vi "Update fgv objectives.vi"(8 "error in (no error)":errorcluster, 11 "Config cluster IN":T1) -> (0 "error out":errorcluster)   [LabVIEW 2017]
uses:
  Typedefs/Calibration config.ctl
  Typedefs/Objective Config.ctl
  Typedefs/Prechirper Cal Config.ctl
  Typedefs/PreChirper constants.ctl
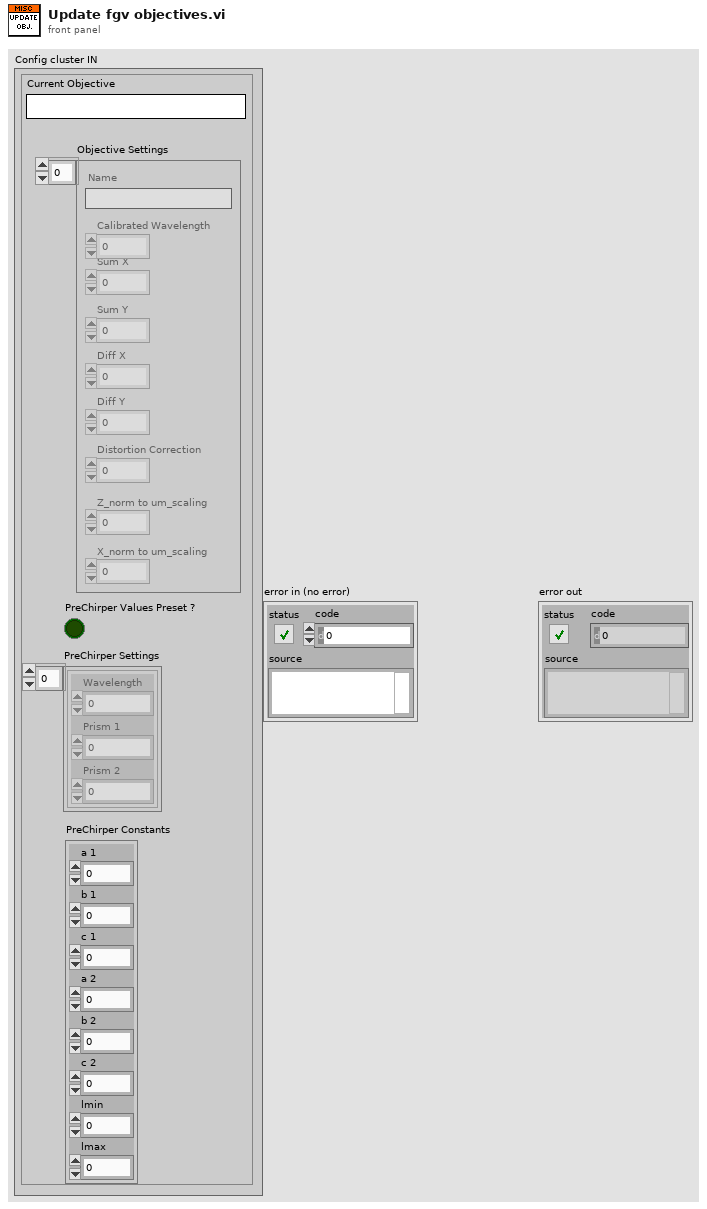
[diagram p1: front panel]
types:
  T1 = typedef "Calibration config.ctl" = cluster{"Current Objective":string, "Objective Settings":T2[], "PreChirper Values Preset ?":bool, "PreChirper Settings":T3[], "PreChirper Constants":T4}
  T2 = typedef "Objective Config.ctl" = cluster{"Name":string, "Sum X":dbl, "Sum Y":dbl, "Diff X":dbl, "Diff Y":dbl, "Distortion Correction":dbl, "Z_norm to um_scaling":dbl, "X_norm to um_scaling":dbl, "Calibrated Wavelength":dbl}
  T3 = typedef "Prechirper Cal Config.ctl" = cluster{"Wavelength":i32, "Prism 1":i32, "Prism 2":i32}
  T4 = typedef "PreChirper constants.ctl" = cluster{"a 1":i32, "b 1":i32, "c 1":i32, "a 2":i32, "b 2":i32, "c 2":i32, "lmin":i32, "lmax":i32}
  T5 = enum16{"Init", "Update Objectives", "Update Current Objective", "Read", "Clear"}
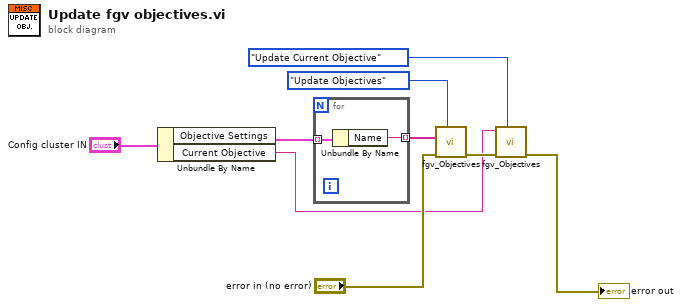
[diagram p0: block diagram]
diagram:
  n1 = Unbundle By Name("Config cluster IN") -> ("Objective Settings"=w8:T2[], "Current Objective"=w2:string)
  n2 = for {
    tunnel: w8 -> [w11] mode=indexing
    tunnel: [w10] -> w5 mode=indexing
    n3 = Unbundle By Name(w11) -> ("Name"=w10:string)
  }
  n4 = call "fgv_Objectives.vi"("Actions"=T5."Update Objectives", "error in (no error)"="error in (no error)", "Objectives"=w5) -> ("error out"=w4:errorcluster)  [unwired: 6 in, 2 out]
  n5 = call "fgv_Objectives.vi"("Actions"=T5."Update Current Objective", "error in (no error)"=w4, "Current Objective"=w2) -> ("error out"=→"error out":errorcluster)  [unwired: 6 in, 2 out]
